vi "subVI_CIR_savetotext_USRP.vi"(0 "file path (dialog if empty)":path, 3 "CIR":dbl[](array[numeric])) -> ()   [LabVIEW 2021]
uses:
  <vilib>/Utility/file.llb/Write Delimited Spreadsheet (DBL).vi
panel:
  out "Array":dbl[](array[numeric])
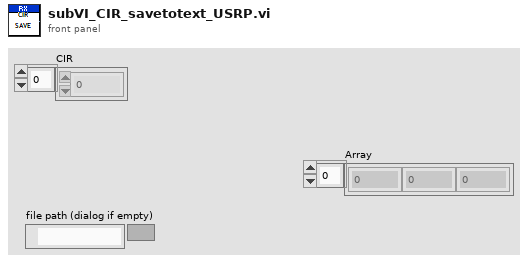
[diagram p1: front panel]
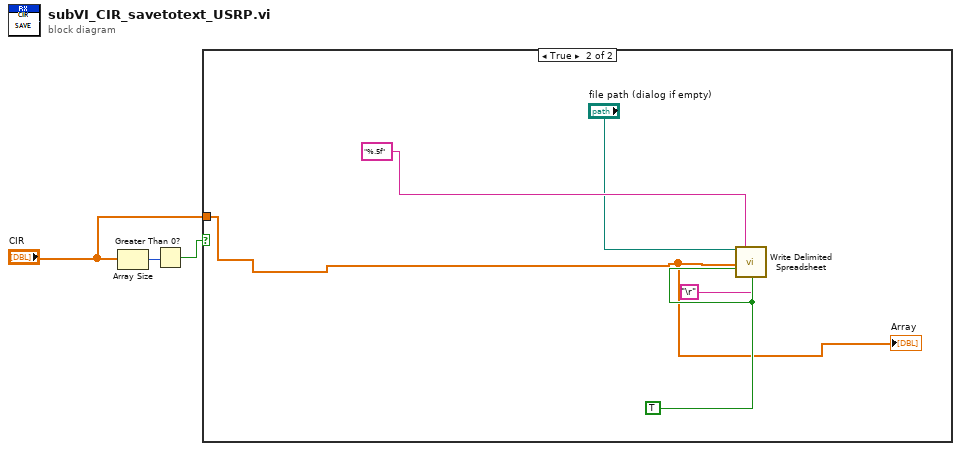
[diagram p0: block diagram]
diagram:
  n1 = Array Size(array="CIR") -> (size(s)=w2:i32)
  n2 = Greater Than 0?(x=w2) -> (x > 0?=w1:bool)
  n3 = case shown="True" w1 {
    tunnel: "CIR" -> [_ w4]
    frame False {
    }
    frame True {
      w7 = TRUE ("transpose? (no:F)")
      n4 = call-poly <vilib>:"Write Delimited Spreadsheet.vi"("file path (dialog if empty)"="file path (dialog if empty)", "format (%.3f)"="%.5f", "1D data"=w4, "append to file? (new file:F)"=w7, "transpose? (no:F)"=w7, "delimiter (\\t)"="\r") -> ()  [unwired: 8 in, 2 out]
      "Array" <- w4
    }
  }
